vi "P4CMD Get Latest Version.vi"(6 "versions":string[](array[string]), 7 "advanced options":variant, 8 "error in (no error)":errorcluster, 9 "retrieval method (file)":T1 items=["file", "directory", "directory (recursive)"], 10 "files":path[](array[path]), 11 "source control reference in":T2) -> (0 "error out":errorcluster, 1 "dialog box cancelled?":bool, 2 "status message":string, 3 "source control reference out":T2)   [LabVIEW 2020, in "NI_SCC_P4CMD.lvlib"]
uses:
  <vilib>/SourceControl/Providers/P4CMD/NI_SCC_P4CMD.lvlib
  <vilib>/SourceControl/sccapi/SCCAPI Refnum.ctl
  <vilib>/SourceControl/sccapi/SCCAPI Get Retrieval Method.ctl
  <vilib>/SourceControl/Providers/P4CMD/P4CMD Operations.ctl
  <vilib>/SourceControl/support/SCCSup Message Strings GLBL.vi
  <vilib>/SourceControl/sccapi/NI_SCC.lvlib
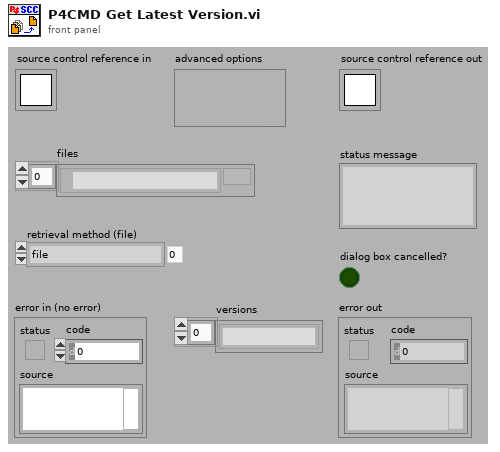
[diagram p1: front panel]
types:
  T1 = typedef "NI_SCC.lvlib/SCCAPI Get Retrieval Method.ctl" = u16
  T2 = typedef "NI_SCC.lvlib/SCCAPI Refnum.ctl" = refnum<k1>
  T3 = typedef "NI_SCC_P4CMD.lvlib/P4CMD Operations.ctl" = enum16{"get all clients", "get all users", "describe changelist", "sync from depot", "open for edit", "submit to depot", "revert", "add to depot", "remove from depot", "print files revisions", "compare client file", "print depot file contents", "list opened files", "get file info", "lock files", "edit changelist spec", "info", "set variables"}
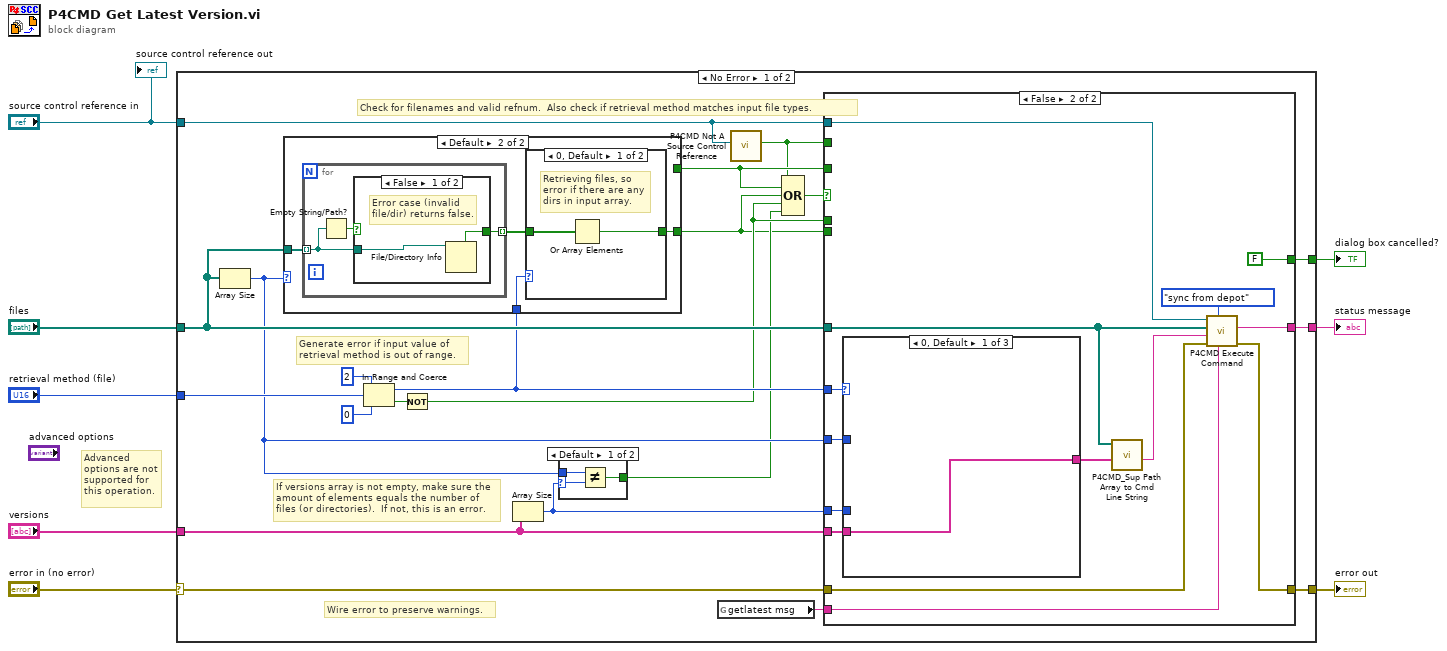
[diagram p0: block diagram]
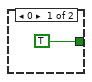
[diagram p3: hidden frame]
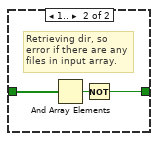
[diagram p4: hidden frame]
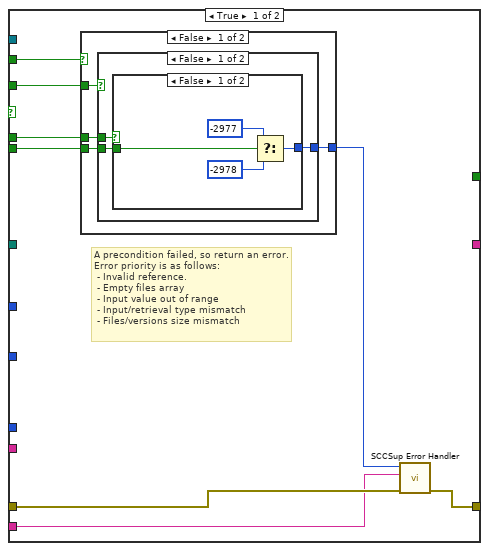
[diagram p6: hidden frame]
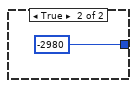
[diagram p7: hidden frame]
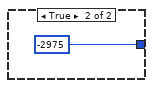
[diagram p8: hidden frame]
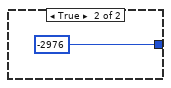
[diagram p9: hidden frame]
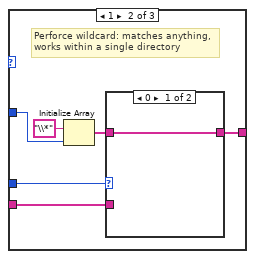
[diagram p10: hidden frame]
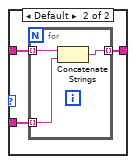
[diagram p11: hidden frame]
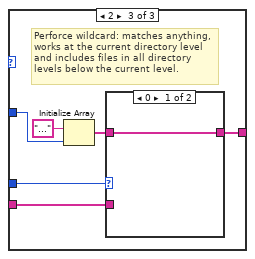
[diagram p12: hidden frame]
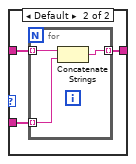
[diagram p13: hidden frame]
diagram:
  # "Advanced options are not supported for this operation."
  n1 = case shown="No Error" "error in (no error)" {
    selector: "error in (no error)" -> [w17 w111]
    tunnel: [w16 w111] -> w7
    tunnel: "source control reference in" -> [w25 _]
    tunnel: [w26 _] -> w5
    tunnel: "files" -> [w23 _]
    tunnel: "retrieval method (file)" -> [w27 _]
    tunnel: [w22 _] -> w2
    tunnel: "versions" -> [w13 _]
    frame No Error {
      # "Generate error if input value of retrieval method is out of range."
      # "If versions array is not empty, make sure the amount of elements equals the number of files (or directories).  If not, this is an error."
      # "Wire error to preserve warnings."
      # "Check for filenames and valid refnum.  Also check if retrieval method matches input file types."
      n2 = Array Size(array=w23) -> (size(s)=w18:i32)
      n3 = In Range and Coerce(upper limit=u16 2, x=w27, lower limit=u16 0) -> (coerced(x)=w19:T1, In Range?=w14:bool)
      n4 = case shown="Default" w18 {
        tunnel: w23 -> [_ w37]
        tunnel: w19 -> [_ w36]
        tunnel: [_ w34] -> w10
        tunnel: [TRUE _] -> w21
        frame 0 {
        }
        frame Default {
          n5 = for {
            tunnel: w37 -> [w43] mode=indexing
            tunnel: [w45] -> w35 mode=indexing
            n6 = Empty String/Path?(string/path=w43) -> (empty?=w44:bool)
            n7 = case shown="False" w44 {
              tunnel: w43 -> [w47 _]
              tunnel: [w46 _] -> w45
              frame False {
                # "Error case (invalid file/dir) returns false."
                n8 = File/Directory Info(path=w47) -> (directory=w46:bool)  [unwired: 1 in, 6 out]
              }
              frame True {
                # "Return false if empty, since file/dir info returns true on empty paths."
              }
            }
          }
          n9 = case shown="0, Default" w36 {
            tunnel: w35 -> [w39 w42]
            tunnel: [w38 w40] -> w34
            frame 0, Default {
              # "Retrieving files, so error if there are any dirs in input array."
              n10 = Or Array Elements(Boolean array=w39) -> (logical OR=w38:bool)
            }
            frame 1.. {
              # "Retrieving dir, so error if there are any files in input array."
              n11 = And Array Elements(Boolean array=w42) -> (logical AND=w41:bool)
              n12 = Not(x=w41) -> (.not. x?=w40:bool)
            }
          }
        }
      }
      n13 = Not(x=w14) -> (.not. x?=w12:bool)
      n14 = Array Size(array=w13) -> (size(s)=w9:i32)
      n15 = case shown="Default" w9 {
        selector: w9 -> [w30 _]
        tunnel: [w32 _] -> w11
        tunnel: w18 -> [w31 _]
        frame Default {
          n16 = Not Equal?(x=w31, y=w30) -> (x != y?=w32:bool)
        }
        frame 0 {
        }
      }
      n17 = global read "SCCSup Message Strings GLBL.vi" "getlatest msg"() -> (w15:string)
      n18 = call <vilib>:"P4CMD Not A Source Control Reference.vi"("source control reference in"=w25) -> ("not a source control reference?"=w20:bool)  [unwired: 9 in, 1 out]
      n19 = Compound Arithmetic op=OR(w20, w21, w10, w12, w11) -> (w24:bool)
      n20 = case shown="False" w24 {
        tunnel: w25 -> [_ w77]
        tunnel: [_ w74] -> w26
        tunnel: w19 -> [_ w82]
        tunnel: w23 -> [_ w76]
        tunnel: w20 -> [w54 _]
        tunnel: w12 -> [w55 _]
        tunnel: [_ FALSE] -> w22
        tunnel: w13 -> [_ w81]
        tunnel: w21 -> [w53 _]
        tunnel: w18 -> [_ w79]
        tunnel: w17 -> [w52 w73]
        tunnel: [w50 w72] -> w16
        tunnel: w15 -> [w49 w71]
        tunnel: w10 -> [w48 _]
        tunnel: w9 -> [_ w70]
        frame True {
          # "A precondition failed, so return an error. \nError priority is as follows:\n - Invalid reference.  \n - Empty files array\n - Input value out of range\n - Input/retrieval type mismatch\n - Files/versions size mismatch"
          n21 = case shown="False" w54 {
            tunnel: [w58 -2976 ("result")] -> w51
            tunnel: w55 -> [w57 _]
            tunnel: w53 -> [w59 _]
            tunnel: w48 -> [w56 _]
            frame False {
              n22 = case shown="False" w59 {
                tunnel: [w62 -2975 ("result")] -> w58
                tunnel: w57 -> [w61 _]
                tunnel: w56 -> [w60 _]
                frame False {
                  n23 = case shown="False" w61 {
                    tunnel: [w66 -2980 ("result")] -> w62
                    tunnel: w60 -> [w63 _]
                    frame False {
                      n24 = Select(t=-2977 ("result"), s=w63, f=-2978 ("result")) -> (s? t:f=w66:i32)
                    }
                    frame True {
                    }
                  }
                }
                frame True {
                }
              }
            }
            frame True {
            }
          }
          n25 = call <vilib>:"SCCSup Error Handler.vi"("error in (no error)"=w52, "operation message"=w49, "scc error code"=w51) -> ("error out"=w50:errorcluster)  [unwired: 8 in]
        }
        frame False {
          n26 = case shown="0, Default" w82 {
            tunnel: w81 -> [w84 w85 w100]
            tunnel: [w84 w88 w99] -> w80
            tunnel: w79 -> [_ w89 w102]
            tunnel: w70 -> [_ w86 w98]
            frame 0, Default {
            }
            frame 1 {
              # "Perforce wildcard: matches anything, works within a single directory"
              n27 = Initialize Array("\\*" ("format string"), w89) -> (w87:string[])
              n28 = case shown="0" w86 {
                tunnel: w87 -> [w91 w94]
                tunnel: w85 -> [_ w93]
                tunnel: [w91 w92] -> w88
                frame 0 {
                }
                frame Default {
                  n29 = for {
                    tunnel: w94 -> [w97] mode=indexing
                    tunnel: w93 -> [w96] mode=indexing
                    tunnel: [w95] -> w92 mode=indexing
                    n30 = Concatenate Strings(w97, w96) -> (w95:string)
                  }
                }
              }
            }
            frame 2 {
              # "Perforce wildcard: matches anything, works at the current directory level and includes files in all directory levels below the current level."
              n31 = Initialize Array("..." ("format string"), w102) -> (w101:string[])
              n32 = case shown="0" w98 {
                tunnel: w101 -> [w104 w107]
                tunnel: w100 -> [_ w106]
                tunnel: [w104 w105] -> w99
                frame 0 {
                }
                frame Default {
                  n33 = for {
                    tunnel: w107 -> [w110] mode=indexing
                    tunnel: w106 -> [w109] mode=indexing
                    tunnel: [w108] -> w105 mode=indexing
                    n34 = Concatenate Strings(w110, w109) -> (w108:string)
                  }
                }
              }
            }
          }
          n35 = call <vilib>:"P4CMD_Sup Path Array to Cmd Line String.vi"("modifiers"=w80, "files"=w76) -> ("string output"=w75:string)  [unwired: 8 in, 1 out]
          n36 = call <vilib>:"P4CMD Execute Command.vi"("operation message"=w71, "p4 operation"=P4CMD_Operations."sync from depot", "error in (no error)"=w73, "input string"=w75, "files"=w76, "source control reference in"=w77) -> ("error out"=w72:errorcluster, "command information"=w74:string)  [unwired: 3 in, 1 out]
        }
      }
    }
    frame Error {
    }
  }
  "error out" <- w7
  "status message" <- w5
  "dialog box cancelled?" <- w2
  "source control reference out" <- "source control reference in"
